vi "Connection.vi"(6 "Parameters":variant, 7 "Timeout":i32=5000, 8 "error in (no error)":errorcluster, 9 "Port":u16=102, 10 "IP Address":string, 11 "PLC_Abstr in":refnum<class "PLC_Abstr.lvclass">) -> (0 "error out":errorcluster, 3 "PLC_Abstr out":refnum<class "PLC_Abstr.lvclass">)   [LabVIEW 2025, in "PLC_Abstr.lvlib" / "PLC_Abstr.lvclass"]
uses:
  PLC_Abstr.lvclass
  PLC_Abstr.lvclass/PLC_Abstr.ctl
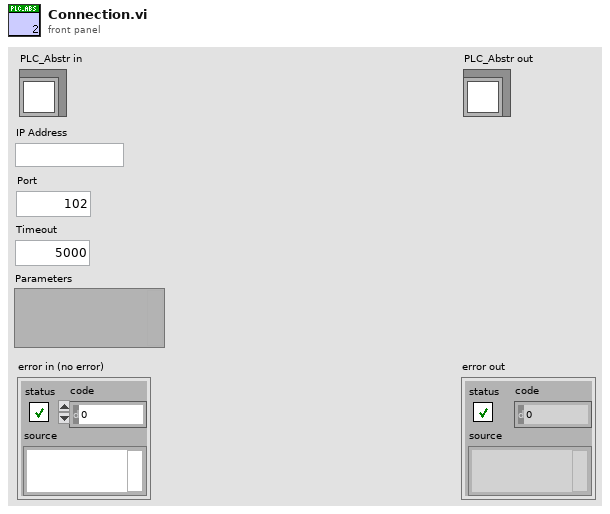
[diagram p1: front panel]
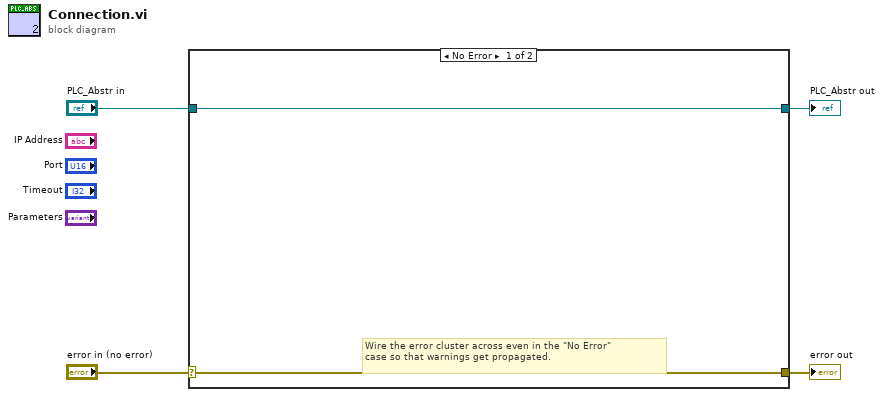
[diagram p0: block diagram]
diagram:
  n1 = case shown="No Error" "error in (no error)" {
    selector: "error in (no error)" -> [w5 w8]
    tunnel: [w5 w8] -> w3
    tunnel: [w6 w7] -> w1
    tunnel: "PLC_Abstr in" -> [w6 w7]
    frame No Error {
      # "Wire the error cluster across even in the \"No Error\"\ncase so that warnings get propagated."
    }
    frame Error {
    }
  }
  "error out" <- w3
  "PLC_Abstr out" <- w1
